vi "SeqCreatePulseArray.vi"(6 "Enabled pulse array 2":T1(array[cluster]), 8 "step #":i32) -> (0 "Pulses":u64[](array[numeric]), 1 "Times":u32[](array[numeric]), 2 "Counts":u8[](array[numeric]), 3 "Triggers":u8[](array[numeric]), 4 "VFG times":dbl[](array[numeric]), 5 "AOs":u8[](array[numeric]))   [LabVIEW 2017]
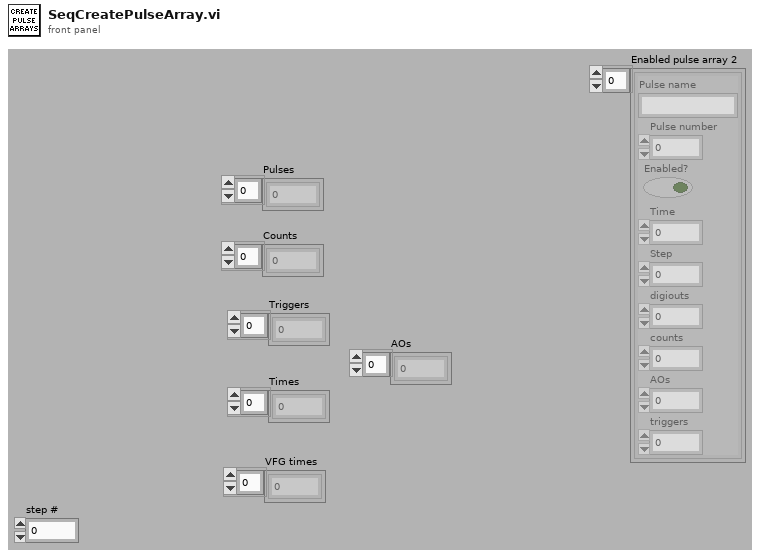
[diagram p1: front panel]
types:
  T1 = cluster{"Pulse name":string, "Pulse number":i32, "Enabled?":bool, "Time":dbl, "Step":dbl, "digiouts":u64, "counts":u8, "AOs":u8, "triggers":u8}[]
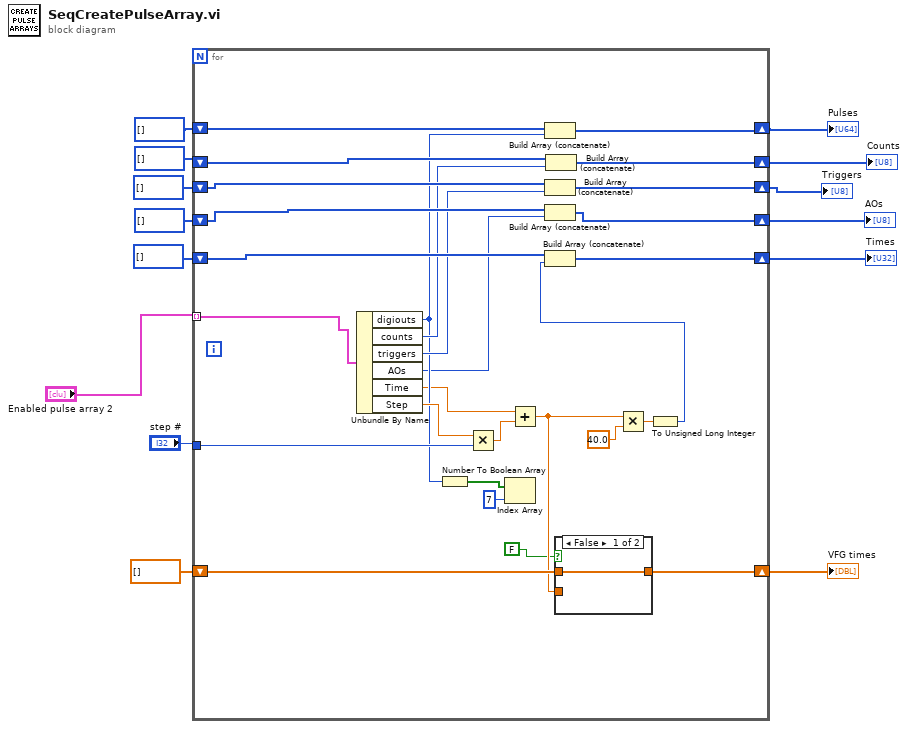
[diagram p0: block diagram]
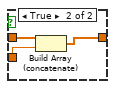
[diagram p2: hidden frame]
diagram:
  n1 = for {
    tunnel: "Enabled pulse array 2" -> [w16] mode=indexing
    shift-right: [w39] -> w5
    shift-left: u8[] [] -> [w42]
    shift-right: [w41] -> w13
    shift-left: u32[] [] -> [w40]
    shift-right: [w38] -> w6
    shift-left: u8[] [] ("Count") -> [w37]
    tunnel: "step #" -> [w36]
    shift-right: [w34] -> w8
    shift-left: dbl[] [] -> [w35]
    shift-right: [w32] -> w4
    shift-left: u64[] [] -> [w33]
    shift-right: [w30] -> w2
    shift-left: u8[] [] -> [w31]
    n2 = Unbundle By Name(w16) -> ("digiouts"=w19:u64, "counts"=w21:u8, "triggers"=w20:u8, "AOs"=w17:u8, "Time"=w18:dbl, "Step"=w22:dbl)
    n3 = Number To Boolean Array(number=w19) -> (Boolean array=w24:bool[])
    n4 = Multiply(x=w22, y=w36) -> (x*y=w29:dbl)
    n5 = Index Array(array=w24, index=7) -> ()  [unwired: 1 out]
    n6 = Add(x=w18, y=w29) -> (x+y=w23:dbl)
    n7 = Build Array (concatenate)(w33, w19) -> (w32:u64[])
    n8 = Build Array (concatenate)(w42, w20) -> (w39:u8[])
    n9 = Build Array (concatenate)(w31, w17) -> (w30:u8[])
    n10 = Build Array (concatenate)(w37, w21) -> (w38:u8[])
    n11 = case shown="False" FALSE {
      tunnel: w35 -> [w43 w45]
      tunnel: w23 -> [_ w46]
      tunnel: [w43 w44] -> w34
      frame False {
      }
      frame True {
        n12 = Build Array (concatenate)(w45, w46) -> (w44:dbl[])
      }
    }
    n13 = Multiply(x=w23, y=40.0) -> (x*y=w27:dbl)
    n14 = To Unsigned Long Integer(number=w27) -> (unsigned 32bit integer=w26:u32)
    n15 = Build Array (concatenate)(w40, w26) -> (w41:u32[])
  }
  "Times" <- w13
  "Counts" <- w6
  "Pulses" <- w4
  "VFG times" <- w8
  "Triggers" <- w5
  "AOs" <- w2
